vi "Парал-рег-класт.vi"(0 "C":bool, 2 "Reset":bool, 3 "Cluster I":T2) -> (1 "Cluster O":T1)   [LabVIEW 2017]
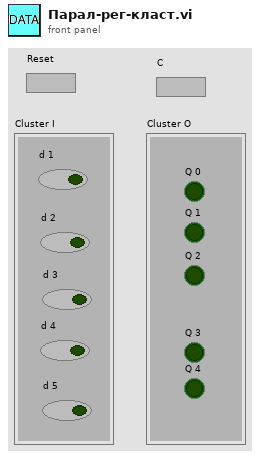
[diagram p1: front panel]
types:
  T1 = cluster{"Q 0":bool, "Q 1":bool, "Q 2":bool, "Q 3":bool, "Q 4":bool}
  T2 = cluster{"d 1":bool, "d 2":bool, "d 3":bool, "d 4":bool, "d 5":bool}
  T3 = cluster{"q":bool, "q":bool, "q":bool, "q":bool, "q":bool}
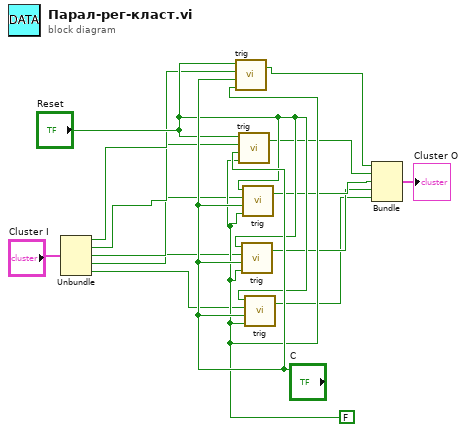
[diagram p0: block diagram]
diagram:
  w13 = FALSE
  n1 = Unbundle("Cluster I") -> ("d 1"=w10:bool, "d 2"=w9:bool, "d 3"=w8:bool, "d 4"=w7:bool, "d 5"=w6:bool)
  n2 = call "trig.vi"("s"=w13, "c"="C", "d"=w10, "r"="Reset") -> ("q"=w5:bool)  [unwired: 1 out]
  n3 = call "trig.vi"("s"=w13, "c"="C", "d"=w9, "r"="Reset") -> ("q"=w4:bool)  [unwired: 1 out]
  n4 = call "trig.vi"("s"=w13, "c"="C", "d"=w7, "r"="Reset") -> ("q"=w2:bool)  [unwired: 1 out]
  n5 = call "trig.vi"("s"=w13, "c"="C", "d"=w8, "r"="Reset") -> ("q"=w3:bool)  [unwired: 1 out]
  n6 = call "trig.vi"("s"=w13, "c"="C", "d"=w6, "r"="Reset") -> ("q"=w1:bool)  [unwired: 1 out]
  n7 = Bundle("q"=w5, "q"=w4, "q"=w3, "q"=w2, "q"=w1) -> (→"Cluster O":T3)  [unwired: 1 in]
